vi "Configure Reference.vi"(7 "Set Reference Method (0: Reference)":u16(ring) items=["Reference", "Input"], 8 "error in (no error)":errorcluster, 9 "Enable Reference Mode (T:Enable)":bool=TRUE, 10 "Reference Value (0.00001)":dbl=1e-05 min=1e-05 max=20000000.0 format="%.5f", 11 "VISA resource name":refnum<visa-resource-name>) -> (0 "error out":errorcluster, 3 "VISA resource name out":refnum<visa-resource-name>)   [LabVIEW 2014, in "BK Precision 5491B.lvlib"]
doc: "Configures and enables reference mode for the primary measurement function.\n\n<b>Note: Reference mode does not apply to secondary measurement function.</b>"
uses:
  <instrlib>/BK Precision 5491B/BK Precision 5491B.lvlib
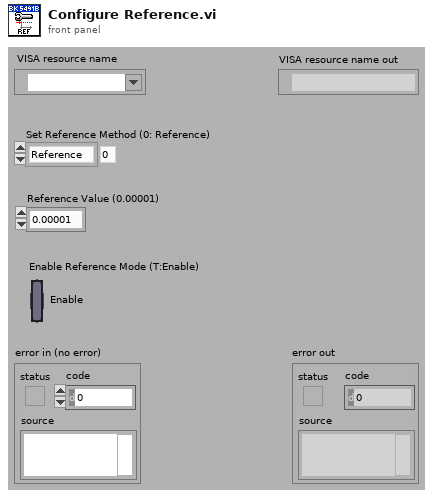
[diagram p1: front panel]
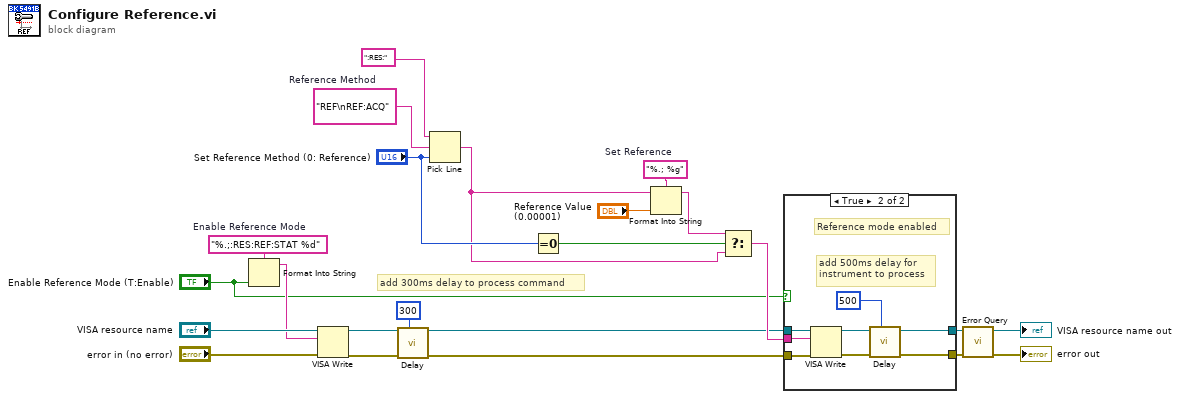
[diagram p0: block diagram]
diagram:
  w11 = "%.;:RES:REF:STAT %d"  # Enable Reference Mode
  w20 = "%.; %g"  # Set Reference
  w21 = "REF\nREF:ACQ"  # Reference Method
  # "add 300ms delay to process command"
  n1 = Format Into String(format string=w11, "Enable Reference Mode (T:Enable)") -> (resulting string=w8:string)  [unwired: 2 in, 1 out]
  n2 = VISA Write(VISA resource name="VISA resource name", write buffer=w8, error in (no error)="error in (no error)") -> (VISA resource name out=w6:refnum<visa-resource-name>, error out=w5:errorcluster)  [unwired: 1 out]
  n3 = call <instrlib>:"Delay.vi"("Delay Time (0)"=u32 300, "error in (no error)"=w5, "VISA resource name"=w6) -> ("error out"=w4:errorcluster, "VISA resource name out"=w3:refnum<visa-resource-name>)  [unwired: 7 in]
  n4 = Pick Line(string ("")=":RES:", multi-line string=w21, line index="Set Reference Method (0: Reference)") -> (output string=w12:string)
  n5 = Equal To 0?(x="Set Reference Method (0: Reference)") -> (x = 0?=w15:bool)
  n6 = Format Into String(format string=w20, initial string=w12, "Reference Value (0.00001)") -> (resulting string=w13:string)  [unwired: 1 in, 1 out]
  n7 = Select(t=w13, s=w15, f=w12) -> (s? t:f=w7:string)
  n8 = case shown="True" "Enable Reference Mode (T:Enable)" {
    tunnel: [w25 w32] -> w19
    tunnel: [w24 w31] -> w18
    tunnel: w7 -> [_ w28]
    tunnel: w4 -> [w24 w27]
    tunnel: w3 -> [w25 w26]
    frame False {
      # "Reference mode\ndisabled"
    }
    frame True {
      # "Reference mode enabled"
      # "add 500ms delay for\ninstrument to process"
      n9 = VISA Write(VISA resource name=w26, write buffer=w28, error in (no error)=w27) -> (VISA resource name out=w33:refnum<visa-resource-name>, error out=w30:errorcluster)  [unwired: 1 out]
      n10 = call <instrlib>:"Delay.vi"("Delay Time (0)"=u32 500, "error in (no error)"=w30, "VISA resource name"=w33) -> ("error out"=w31:errorcluster, "VISA resource name out"=w32:refnum<visa-resource-name>)  [unwired: 7 in]
    }
  }
  n11 = call <instrlib>:"Error Query.vi"("error in (no error)"=w18, "VISA resource name"=w19) -> ("error out"=→"error out":errorcluster, "VISA resource name out"=→"VISA resource name out":refnum<visa-resource-name>)  [unwired: 7 in, 1 out]
